vi "3D Polynomial Fit.vi"(7 "3D Graph ref":refnum<vi>, 8 "error in":errorcluster, 9 "Highest order":i32=2 min=0, 11 "X,Y,,Z data":dbl[][](array[numeric])=[[0.0, 0.0, 14.0], [40.0, 0.0, 13.0], [80.0, 0.0, 10.0], [0.0, 40.0, 14.0], [40.0, 40.0, 19.0], [80.0, 40.0, 16.0], [0.0, 80.0, 14.0], [40.0, 80.0, 20.0], [80.0, 80.0, 21.0]] format="%.2f") -> (0 "error out":errorcluster, 1 "Best Fit Z":dbl[](array[numeric]) format="%.2f", 2 "Coefficients":dbl[](array[numeric]) format="%.3e", 3 "terms":string[](array[string]), 4 "Time elapsed (ms)":u32)   [LabVIEW 2009]
doc: "This .vi fits using least squares the input (X,Y,Z) coordinates (can be unordered) using a 3D polynomial : Z = A1 + A2x + A3y + A4xy + A5x^2 + A6y^2 .....\n\nHighest order = 0 (level plane)\nHighest order = 1 (sloped plane)\nHighest order = 2 (parabola)\n....\n\nConnecting a reference to the 3D graph ref control will allow you to plot the data and fit together on the same plot. Copy the 3D Graph on this front panel for good results."
uses:
  <vilib>/Analysis/6fits.llb/General Linear Fit Algorithm.ctl
  <vilib>/Native 3D Graph/xcontrol/3DPC_SurfacePlot.xctl
  <vilib>/Analysis/NI_AALPro.lvlib
panel:
  out "3D Graph":refnum<class "Base Datatype.lvclass">[](xcontrol)
  out "# of Coefficients":i32
  in  "algorithm":T1=4 items=["SVD", "Givens", "Givens2", "Householder", "LU Decomposition", "Cholesky", "SVD for Rank Deficient H"]
  out "Formula from fit":string
  out "MSE":dbl format="%.5f"
  # "Z"
  # "X"
  # "Y"
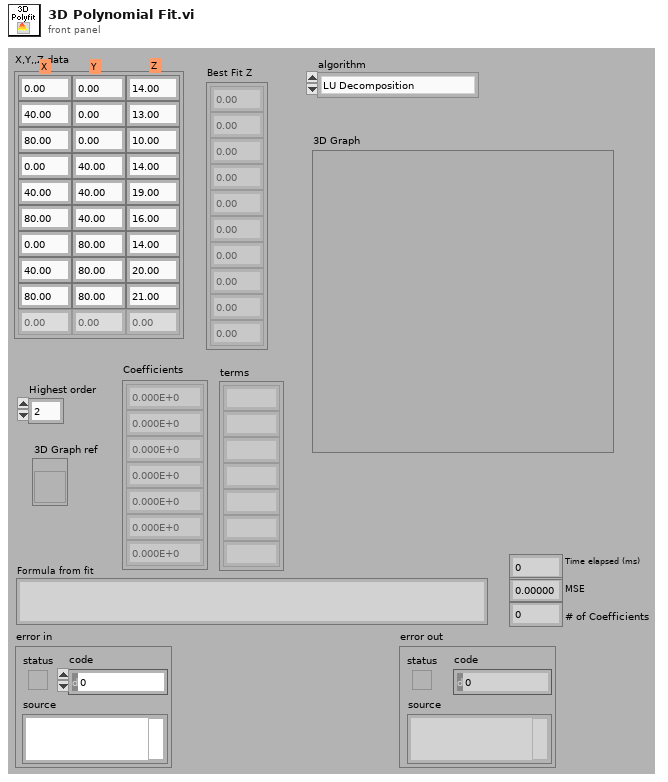
[diagram p1: front panel]
types:
  T1 = typedef "NI_AALPro.lvlib/General Linear Fit Algorithm.ctl" = u16
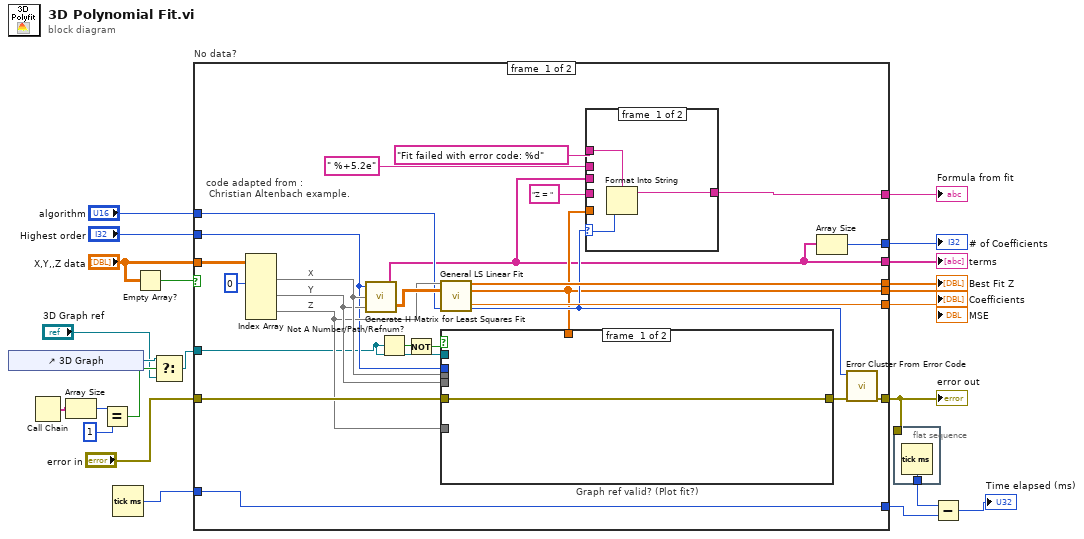
[diagram p0: block diagram]
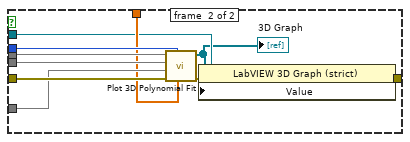
[diagram p2: hidden frame]
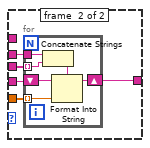
[diagram p3: hidden frame]
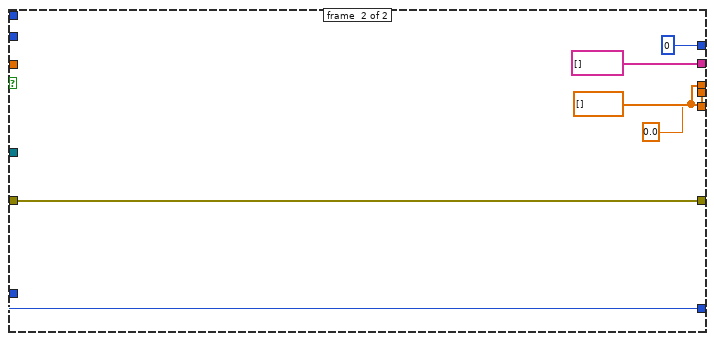
[diagram p4: hidden frame]
diagram:
  n1 = control-ref of="3D Graph"() -> (w8:refnum<vi>)
  n2 = Call Chain() -> (call chain=w12:string[])
  n3 = Array Size(array=w12) -> (size(s)=w11:i32)
  n4 = Equal?(x=w11, y=1) -> (x = y?=w9:bool)
  n5 = Tick Count (ms)() -> (millisecond timer value=w5:u32)
  n6 = Empty Array?(array="X,Y,,Z data") -> (empty?=w16:bool)
  n7 = Select(t=w8, s=w9, f="3D Graph ref") -> (s? t:f=w6:refnum<vi>)
  n8 = case "No data?" shown="False" w16 {
    tunnel: [w48 0.0 ("mse")] -> w23
    tunnel: [w47 _] -> w22
    tunnel: [w27 string[] [] ("[terms]")] -> w21
    tunnel: [w44 0] -> w20
    tunnel: [w43 w77] -> w19
    tunnel: [w34 w74] -> w1
    tunnel: [w30 w77] -> w18
    tunnel: "X,Y,,Z data" -> [w37 _]
    tunnel: [w33 w75] -> w3
    tunnel: w5 -> [w33 w75]
    tunnel: "error in" -> [w32 w74]
    tunnel: "algorithm" -> [w29 _]
    tunnel: "Highest order" -> [w28 _]
    tunnel: w6 -> [w25 _]
    frame #0 {
      # "Z"
      # "Y"
      # "X"
      # "code adapted from : \n Christian Altenbach example."
      n9 = Index Array(array=w37, index (col) #1=0 ("disabled index (col)")) -> (element #1=w39:dbl[], element #2=w38:dbl[], element #3=w31:dbl[])  [unwired: 5 in]
      n10 = call "Generate H Matrix for Least Squares Fit.vi"("[Y]"=w38, "[X]"=w39, "Highest order"=w28) -> ("H"=w41:dbl[][], "[terms]"=w27:string[])
      n11 = Not A Number/Path/Refnum?(number/path/refnum=w25) -> (NaN/Path/Refnum?=w26:bool)
      n12 = Not(x=w26) -> (.not. x?=w24:bool)
      n13 = call <vilib>:"General LS Linear Fit.vi"("Y"=w31, "H"=w41, "algorithm"=w29) -> ("Best Fit"=w43:dbl[], "Coefficients"=w30:dbl[], "mse"=w48:dbl, "error"=w36:i32)  [unwired: 2 in, 7 out]
      n14 = case "Graph ref valid? (Plot fit?)" shown="True" w24 {
        tunnel: w31 -> [_ w56]
        tunnel: w32 -> [w49 w59]
        tunnel: w39 -> [_ w58]
        tunnel: w38 -> [_ w57]
        tunnel: [w49 w51] -> w35
        tunnel: w28 -> [_ w55]
        tunnel: w30 -> [_ w54]
        tunnel: w25 -> [_ w52]
        frame #0 {
        }
        frame #1 {
          n15 = call "Plot 3D Polynomial Fit.vi"("Coefficients"=w54, "Highest order"=w55, "error in"=w59, "Z"=w56, "Y"=w57, "X"=w58) -> ("error out"=w53:errorcluster, "3D Graph"=w50:refnum<class "Base Datatype.lvclass">[])  [unwired: 1 in, 3 out]
          "3D Graph" <- w50
          n16 = property class="LabVIEW 3D Graph (strict)"(reference=w52, error in=w53, "Value"=w50) -> (error out=w51:errorcluster)  [unwired: 1 out]
        }
      }
      n17 = case shown="0" w36 {
        selector: w36 -> [w62 _]
        tunnel: w30 -> [_ w66]
        tunnel: [w61 w67] -> w47
        tunnel: "Fit failed with error code: %d" ("format string") -> [w60 _]
        tunnel: w27 -> [_ w65]
        tunnel: " %+5.2e" ("format string") -> [_ w64]
        tunnel: "Z = " -> [_ w63]
        frame #0 {
          n18 = Format Into String(format string=w60, w62) -> (resulting string=w61:string)  [unwired: 2 in, 1 out]
        }
        frame #1 {
          n19 = for {
            shift-right: [w73] -> w67
            shift-left: w63 -> [w72]
            tunnel: w66 -> [w71] mode=indexing
            tunnel: w65 -> [w70] mode=indexing
            tunnel: w64 -> [w68]
            n20 = Concatenate Strings(w68, w70) -> (w69:string)
            n21 = Format Into String(format string=w69, initial string=w72, w71) -> (resulting string=w73:string)  [unwired: 1 in, 1 out]
          }
        }
      }
      n22 = Array Size(array=w27) -> (size(s)=w44:i32)
      n23 = call <vilib>:"Error Cluster From Error Code.vi"("error in (no error)"=w35, "error code (0)"=w36) -> ("error out"=w34:errorcluster)  [unwired: 1 in, 6 out]
    }
    frame #1 {
      w77 = dbl[] [] ("Best Fit")
    }
  }
  "Coefficients" <- w18
  "Best Fit Z" <- w19
  "MSE" <- w23
  "Formula from fit" <- w22
  "# of Coefficients" <- w20
  "terms" <- w21
  "error out" <- w1
  n24 = flat-sequence {
    tunnel: [w80] -> w4
    tunnel: w1 -> [_]
    frame #0 {
      n25 = Tick Count (ms)() -> (millisecond timer value=w80:u32)
    }
  }
  n26 = Subtract(x=w4, y=w3) -> (x-y=→"Time elapsed (ms)":u32)
